vi "CreateParser.vi"(8 "error in (no error)":errorcluster, 10 "PythonModuleDirectory":path, 11 "ArgumentParser in":refnum<class "ArgumentParser.lvclass">) -> (0 "error out":errorcluster, 3 "ArgumentParser out":refnum<class "ArgumentParser.lvclass">)   [LabVIEW 2022 SP3, in "ArgumentParser.lvlib" / "ArgumentParser.lvclass"]
uses:
  ArgumentParser.lvclass
  ArgumentParser.lvclass/ArgumentParser.ctl
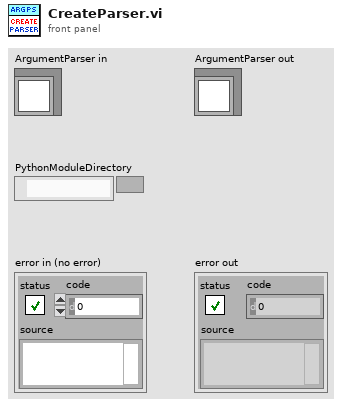
[diagram p1: front panel]
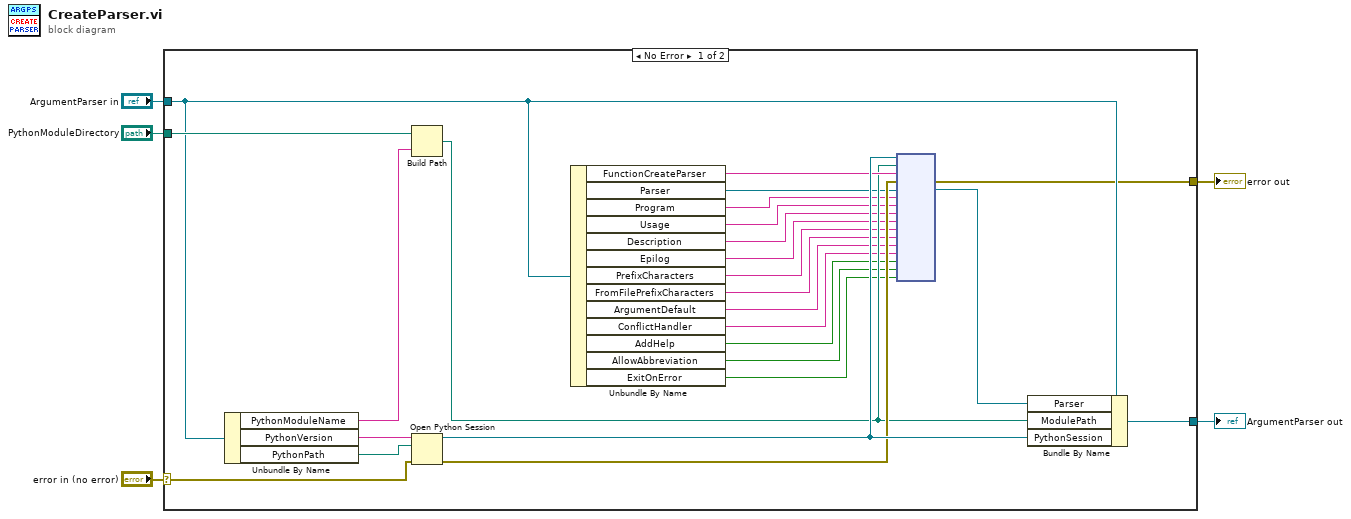
[diagram p0: block diagram]
diagram:
  n1 = case shown="No Error" "error in (no error)" {
    selector: "error in (no error)" -> [w6 w32]
    tunnel: [w20 w32] -> w4
    tunnel: [w28 w31] -> w2
    tunnel: "ArgumentParser in" -> [w23 w31]
    tunnel: "PythonModuleDirectory" -> [w26 _]
    frame No Error {
      n2 = Unbundle By Name(w23) -> ("PythonModuleName"=w25:string, "PythonVersion"=w30:string, "PythonPath"=w29:path)
      n3 = Build Path(base path=w26, name or relative path=w25) -> (appended path=w21:path)
      n4 = Open Python Session(python version=w30, python path=w29, 3:w6) -> (session out=w27:refnum<k35>, error out=w24:errorcluster)
      n5 = Unbundle By Name(w23) -> ("FunctionCreateParser"=w22:string, "Parser"=w19:refnum<k38>, "Program"=w17:string, "Usage"=w16:string, "Description"=w15:string, "Epilog"=w14:string, "PrefixCharacters"=w13:string, "FromFilePrefixCharacters"=w12:string, "ArgumentDefault"=w11:string, "ConflictHandler"=w10:string, "AddHelp"=w9:bool, "AllowAbbreviation"=w8:bool, "ExitOnError"=w7:bool)
      n6 = node(w27, w21, w22, w24, w19, w17, w16, w15, w14, w13, w12, w11, w10, w9, w8, w7) -> (w20:errorcluster, w18:refnum<k38>)  [unwired: 11 in, 3 out]
      n7 = Bundle By Name(cluster=w23, "Parser"=w18, "ModulePath"=w21, "PythonSession"=w27) -> (w28:refnum<class "ArgumentParser.lvclass">)
    }
    frame Error {
    }
  }
  "error out" <- w4
  "ArgumentParser out" <- w2
